vi "default_id.vi"(1 "id (unnamed)":string) -> (0 "String":string)   [LabVIEW 2019, in "Lookup API.lvlib" / "Mapped Lookup.lvclass"]
uses:
  Mapped Lookup.lvclass
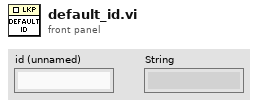
[diagram p1: front panel]
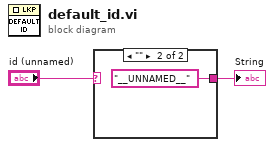
[diagram p0: block diagram]
diagram:
  n1 = case shown="\"\"" "id (unnamed)" {
    selector: "id (unnamed)" -> [w3 _]
    tunnel: [w3 "__UNNAMED__"] -> w2
    frame Default {
    }
    frame "" {
    }
  }
  "String" <- w2
